vi "get update settings.vi"(7 "settings DB OP":enum16{"Get settings", "Update settings"}(ring), 8 "error in (no error)":errorcluster, 11 "REF in":T1) -> (0 "error out":errorcluster, 2 "success?":bool, 3 "REF out":T1)   [LabVIEW 2024]
uses:
  CTRLS/REF.ctl
  CTRLS/Main Tabs.ctl
  CTRLS/Open Batch Data.ctl
  CTRLS/DM_Data.ctl
  CTRLS/run statistics.ctl
  CTRLS/System settings.ctl
  CTRLS/Printer Message settings.ctl
  CTRLS/DB operation Selector.ctl
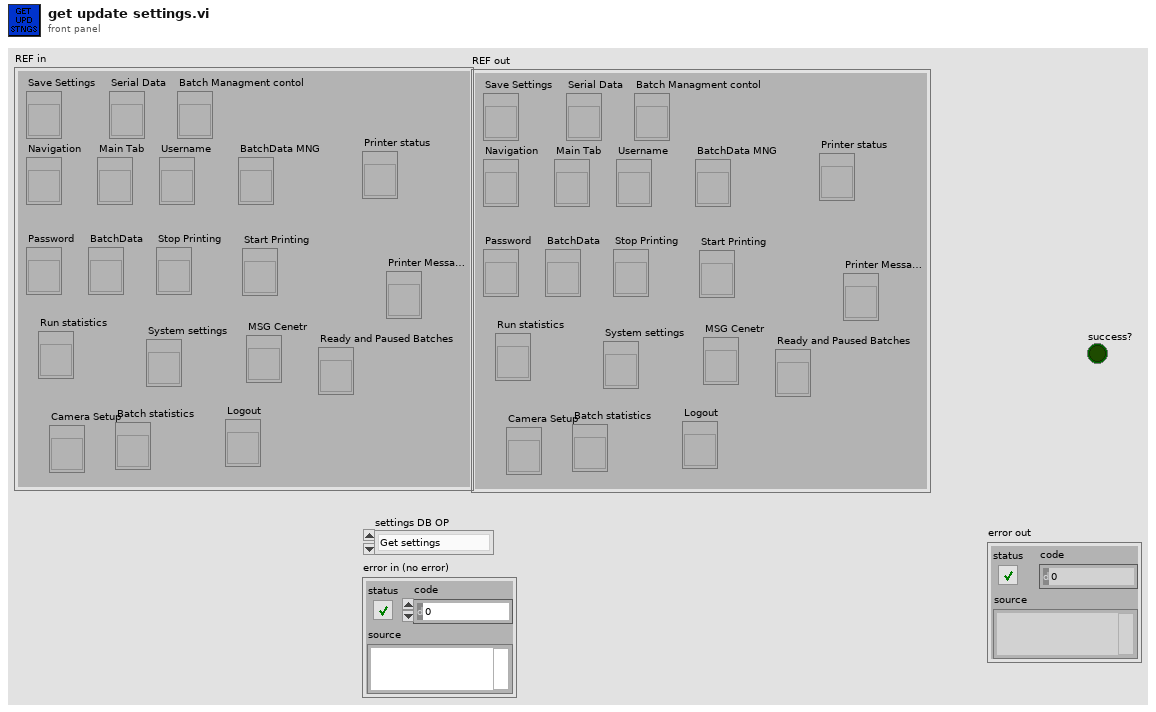
[diagram p1: front panel]
types:
  T1 = typedef "REF.ctl" = cluster{"Save Settings":refnum<vi>, "Navigation":refnum<vi>, "Main Tab":refnum<vi>, "Password":refnum<vi>, "BatchData":refnum<vi>, "Serial Data":refnum<vi>, "Username":refnum<vi>, "Stop Printing":refnum<vi>, "Run statistics":refnum<vi>, "System settings":refnum<vi>, "Batch Managment contol":refnum<vi>, "Start Printing":refnum<vi>, "BatchData MNG":refnum<vi>, "MSG Cenetr":refnum<vi>, "Printer status":refnum<vi>, "Printer Message Config":refnum<vi>, "Ready and Paused Batches":refnum<vi>, "Camera Setup":refnum<vi>, "Batch statistics":refnum<vi>, "Logout":refnum<vi>}
  T2 = typedef "Printer Message settings.ctl" = cluster{"Layout File":string, "Date Separator":string, "OCR Font":string, "Variable Data":string, "Date Layout":string}
  T3 = typedef "DB operation Selector.ctl" = enum16{"Select", "Insert", "Update", "Execute select Query", "Execute update query"}
  T4 = typedef "NI_Database_API.lvlib/Conn ObjectReference.ctl" = refnum<k1>
  T5 = typedef "System settings.ctl" = cluster{"Machine IP":string, "Camera IP":string, "Printer IP":string, "Scanner settings":string, "Server Path":path, "Sending Port":u32, "Recieveing Port":u32}
  T6 = cluster{"Printer IP":string, "Camera IP":string, string, string, "Machine IP":string, string, "xml string":string}
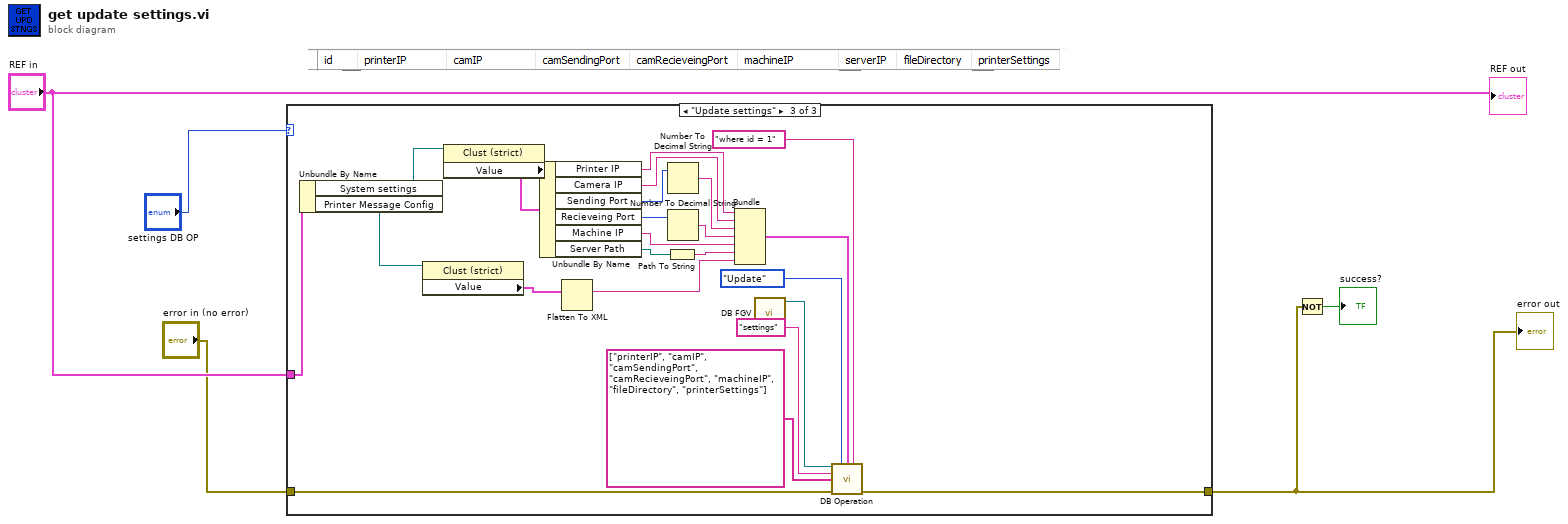
[diagram p0: block diagram]
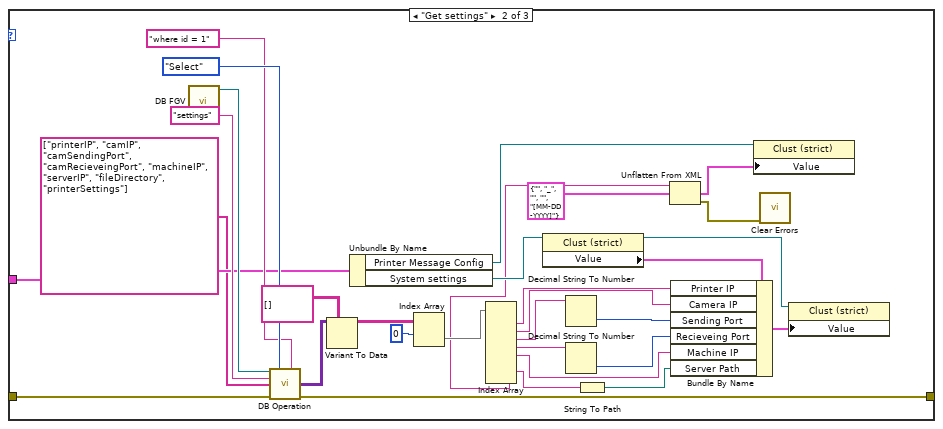
[diagram p3: hidden frame]
diagram:
  n1 = case shown="\"Update settings\"" "settings DB OP" {
    tunnel: "REF in" -> [_ w33 w56]
    tunnel: [w6 w12 w42] -> w2
    tunnel: "error in (no error)" -> [w6 w13 w41]
    frame Default {
    }
    frame "Get settings" {
      n2 = call "DB FGV.vi"() -> ("DB ref"=w36:T4)  [unwired: 11 in]
      n3 = call "DB Operation.vi"("connection reference"=w36, "DB Op Selector"=DB_operation_Selector."Select", "Condition"="where id = 1", "table"="settings", "columns"=string[] ["printerIP", "camIP", "camSendingPort", "camRecieveingPort", "machineIP", "serverIP", "fileDirectory", "printerSettings"], "error in (no error)"=w13) -> ("data out"=w27:variant[][], "error out"=w12:errorcluster)  [unwired: 7 in, 1 out]
      n4 = Variant To Data(type=string[][] [], Variant=w27) -> (data=w26:string[][])  [unwired: 1 in, 1 out]
      n5 = Unbundle By Name(w33) -> ("Printer Message Config"=w11:refnum<vi>, "System settings"=w32:refnum<vi>)
      n6 = Index Array(array=w26, index (row)=0) -> (element=w24:string[])  [unwired: 1 in]
      n7 = Index Array(array=w24) -> (element #1=w22:string, element #2=w21:string, element #3=w19:string, element #4=w18:string, element #5=w16:string, element #7=w15:string, element #8=w10:string)  [unwired: 8 in, 1 out]
      n8 = property class="Clust (strict)"(reference=w32) -> (reference out=w30:refnum<vi>, "Value"=w31:T5)  [unwired: 1 in, 1 out]
      n9 = Decimal String To Number(string=w19) -> (number=w20:i32)  [unwired: 2 in, 1 out]
      n10 = Decimal String To Number(string=w18) -> (number=w17:i32)  [unwired: 2 in, 1 out]
      n11 = String To Path(string=w15) -> (path=w14:path)
      n12 = Unflatten From XML(xml string=w10, type=T2 {"Layout File"="", "Date Separator"="_", "OCR Font"="", "Variable Data"="", "Date Layout"="[MM-DD-YYYY]"} ("Value")) -> (value=w8:T2, error out=w7:errorcluster)  [unwired: 1 in]
      n13 = Bundle By Name(cluster=w31, "Printer IP"=w22, "Camera IP"=w21, "Sending Port"=w20, "Recieveing Port"=w17, "Machine IP"=w16, "Server Path"=w14) -> (w29:T5)
      n14 = property class="Clust (strict)"(reference=w11, "Value"=w8) -> ()  [unwired: 1 in, 2 out]
      n15 = call <vilib>:"Clear Errors.vi"("error in (no error)"=w7) -> ()  [unwired: 5 in, 2 out]
      n16 = property class="Clust (strict)"(reference=w30, "Value"=w29) -> ()  [unwired: 1 in, 2 out]
    }
    frame "Update settings" {
      n17 = Unbundle By Name(w56) -> ("System settings"=w55:refnum<vi>, "Printer Message Config"=w40:refnum<vi>)
      n18 = property class="Clust (strict)"(reference=w40) -> ("Value"=w39:T2)  [unwired: 1 in, 2 out]
      n19 = property class="Clust (strict)"(reference=w55) -> ("Value"=w53:T5)  [unwired: 1 in, 2 out]
      n20 = Unbundle By Name(w53) -> ("Printer IP"=w49:string, "Camera IP"=w48:string, "Sending Port"=w51:u32, "Recieveing Port"=w50:u32, "Machine IP"=w45:string, "Server Path"=w52:path)
      n21 = Flatten To XML(6:w39) -> (2:w38:string)
      n22 = Path To String(path=w52) -> (string=w44:string)
      n23 = Number To Decimal String(number=w51) -> (decimal integer string=w47:string)  [unwired: 1 in]
      n24 = Number To Decimal String(number=w50) -> (decimal integer string=w46:string)  [unwired: 1 in]
      n25 = Bundle("Printer IP"=w49, "Camera IP"=w48, w47, w46, "Machine IP"=w45, w44, "xml string"=w38) -> (w43:T6)  [unwired: 1 in]
      n26 = call "DB FGV.vi"() -> ("DB ref"=w59:T4)  [unwired: 11 in]
      n27 = call "DB Operation.vi"("connection reference"=w59, "DB Op Selector"=DB_operation_Selector."Update", "data"=w43, "Condition"="where id = 1", "table"="settings", "columns"=string[] ["printerIP", "camIP", "camSendingPort", "camRecieveingPort", "machineIP", "fileDirectory", "printerSettings"], "error in (no error)"=w41) -> ("error out"=w42:errorcluster)  [unwired: 6 in, 2 out]
    }
  }
  "error out" <- w2
  n28 = Not(x=w2) -> (.not. x?=→"success?":bool)
  "REF out" <- "REF in"
